vi "Find Child Attributes.vi"(10 "UID":string, 11 "Actor in":refnum<class "Actor.lvclass">) -> (0 "Error out":errorcluster, 2 "Child Attributes":refnum<class "Attributes.lvclass">)   [LabVIEW 2025, in "jettl.lvlib" / "Actor.lvclass"]
uses:
  Actor.lvclass
  Attributes/Attributes/Attributes.lvclass
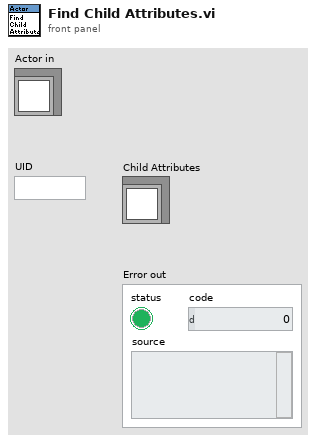
[diagram p1: front panel]
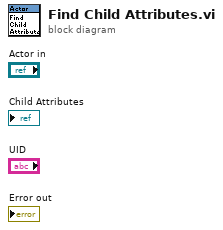
[diagram p0: block diagram]
diagram:
